vi "Scan action.vi"(8 "error in (no error)":errorcluster, 11 "SweepControl in":refnum<class "Sweep Control.lvclass">) -> (0 "error out":errorcluster, 1 "Stop?":bool, 3 "SweepControl out":refnum<class "Sweep Control.lvclass">)   [LabVIEW 2019, in "Sweep Control.lvclass"]
uses:
  Sweep Control.lvclass
  Sweep Control.lvclass/Sweep Control.ctl
  <userlib>/LevyLab/Transport/Transport/Transport.lvclass/Transport.ctl
  <userlib>/LevyLab/Instrument Framework/Instrument Types/Cryostat/Typedefs/Magnet Mode--Enum.ctl
  <userlib>/LevyLab/Transport/Control Experiment/Control Experiment.lvclass/Control Experiment.ctl
  <userlib>/LevyLab/Transport/Transport/Transport.lvclass
  <userlib>/LevyLab/Transport/Control Experiment/Control Experiment.lvclass
  <userlib>/LevyLab/Instrument Framework/Instrument Types/Lockin/Instrument.LockinAPI.lvclass
  <userlib>/LevyLab/Instrument Framework/Instrument Types/Cryostat/Instrument.Cryostat.lvclass
  <userlib>/LevyLab/Instrument Framework/Instrument Types/Strain/Instrument.Strain.lvclass
  <userlib>/LevyLab/Instrument Framework/Instrument Types/Delay Line/Instrument.DelayLine.lvclass
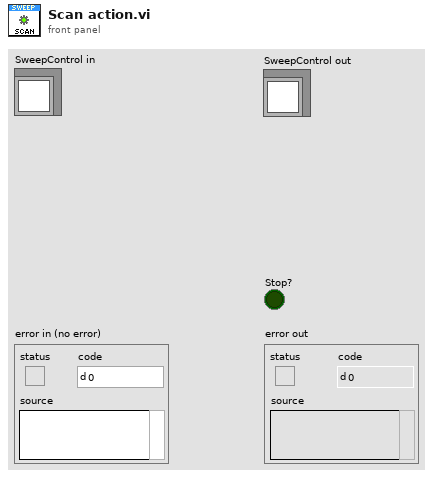
[diagram p1: front panel]
types:
  T1 = typedef "Sweep Control.lvclass/Cluster - Sweep Control.ctl" = cluster{"Start":dbl, "End":dbl, "Step":dbl, "Rate":dbl, "wait (ms/mK)":u32, "Address":string, "Priority":T2, "Scan name":T3, "Post Actions":T4[], "channel":i32}
  T2 = typedef "Sweep Control.lvclass/Enum - Priority.ctl" = enum16{"Priority 0", "Priority 1", "Priority 2", "Priority 3", "Priority 4", "Priority 5"}
  T3 = typedef "Sweep Control.lvclass/Enum - Action.ctl" = enum16{"OFF", "time", "Lockin Amplitude", "Lockin Frequency", "Lockin Bias", "Delay", "Strain", "DAQ Bias", "Magnet Field", "Temperature", "MW f1", "MW f2", "MW Amplitude1", "MW Amplitude2"}
  T4 = typedef "Sweep Control.lvclass/Enum - PostAction.ctl" = enum16{"Do Nothing", "Wait (time)", "Wait (Temperature)", "Wait (<T ; B sweep)", "Wait (Magnet)"}
  T5 = typedef "Sweep Control.lvclass/ScanParamters.ctl" = T6[]
  T6 = typedef "Sweep Control.lvclass/Cluster - ScanParamters.ctl" = cluster{"Start":dbl, "End":dbl, "Step":dbl, "Rate":dbl, "Waveform type":enum16{"linear", "triangle", "power"}, "wait (ms or K)":dbl, "Address":string, "channel":i32}
  T7 = typedef "Sweep Control.lvclass/ScanControl.ctl" = T8[]
  T8 = typedef "Sweep Control.lvclass/Cluster - ScanControl.ctl" = cluster{"Priority":T2, "Scan name":T3}
  T9 = typedef "Control Experiment.lvclass/Instrument Classes--cluster.ctl" = cluster{"DAQ":refnum<class "Instrument.LockinAPI.lvclass">, "Amplifier":refnum<class "Instrument.Amplifier.lvclass">, "Temperature":refnum<class "Instrument.Cryostat.lvclass">, "Magnet":refnum<class "Instrument.Cryostat.lvclass">, "Rotator":refnum<class "Instrument.Cryostat.lvclass">, "Level":refnum<class "Instrument.Cryostat.lvclass">, "Capacitance":refnum<class "Instrument.CBridge.lvclass">, "Delay Line":refnum<class "Instrument.DelayLine.lvclass">, "Strain Cell":refnum<class "Instrument.Strain.lvclass">, "VNA":refnum<class "Instrument.VNA.lvclass">, "Source":refnum<class "Instrument.VSource.lvclass">}
  T10 = typedef "Instrument.Cryostat.lvclass/Magnet Mode--Enum.ctl" = enum16{"Persistent", "Driven"}
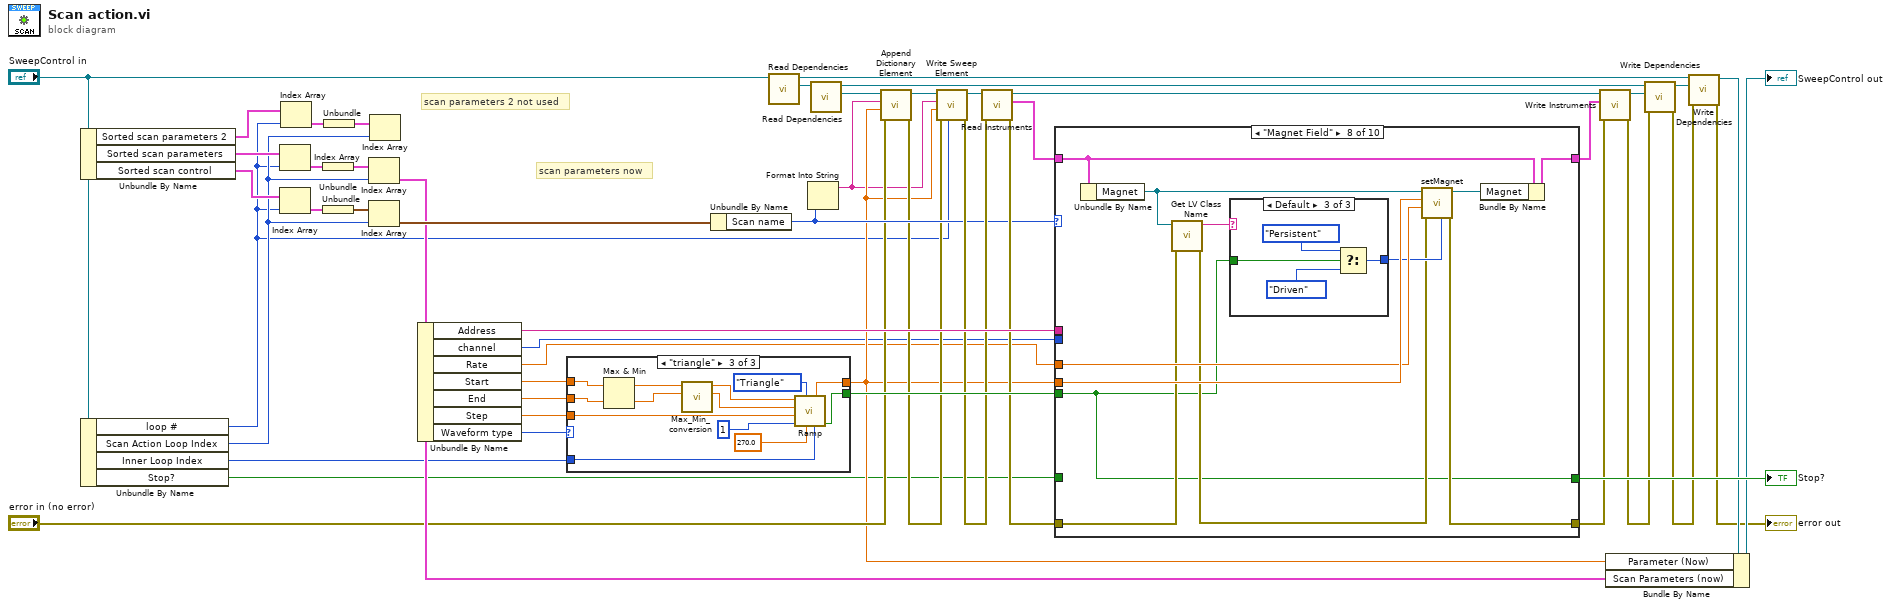
[diagram p0: block diagram]
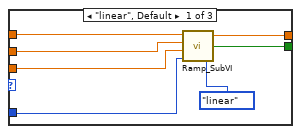
[diagram p2: hidden frame]
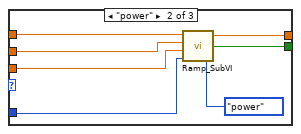
[diagram p3: hidden frame]
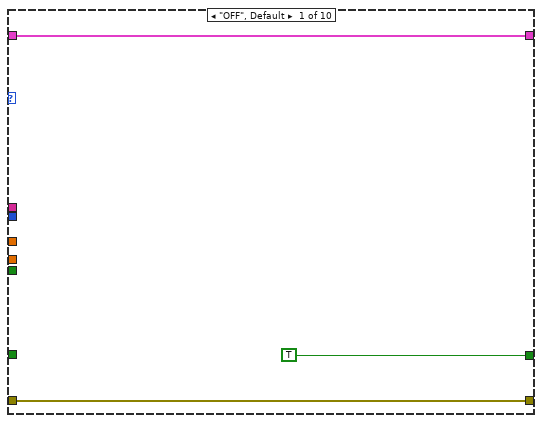
[diagram p4: hidden frame]
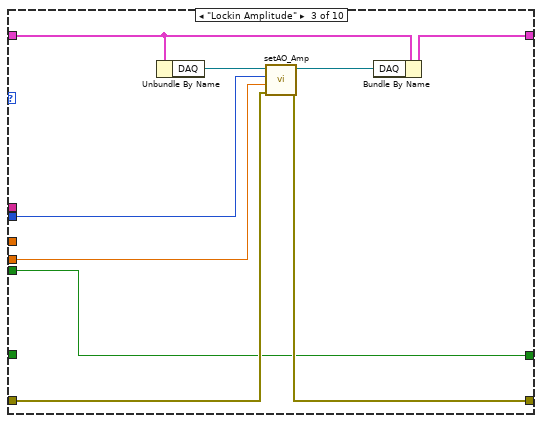
[diagram p6: hidden frame]
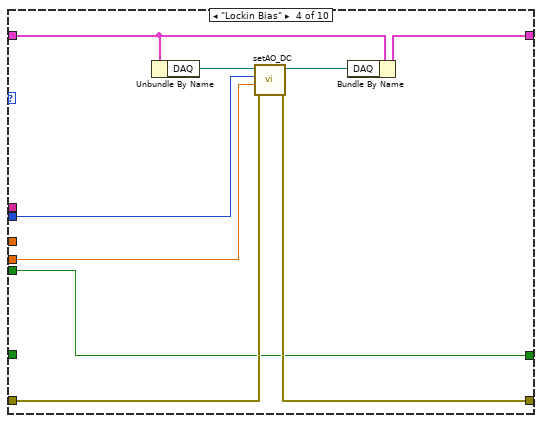
[diagram p7: hidden frame]
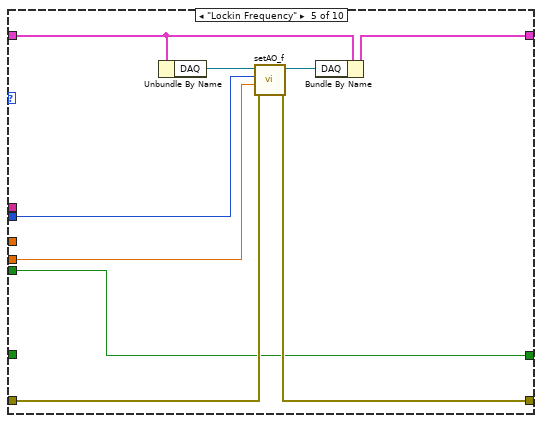
[diagram p8: hidden frame]
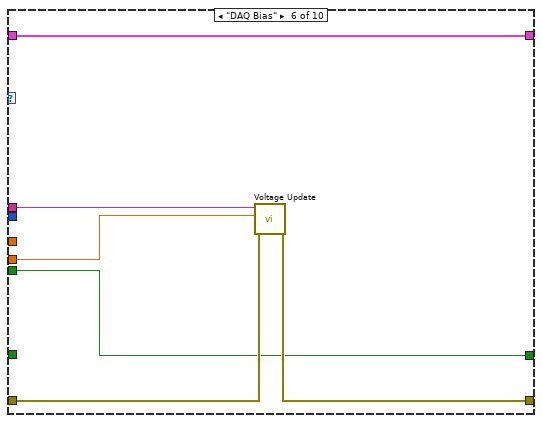
[diagram p9: hidden frame]
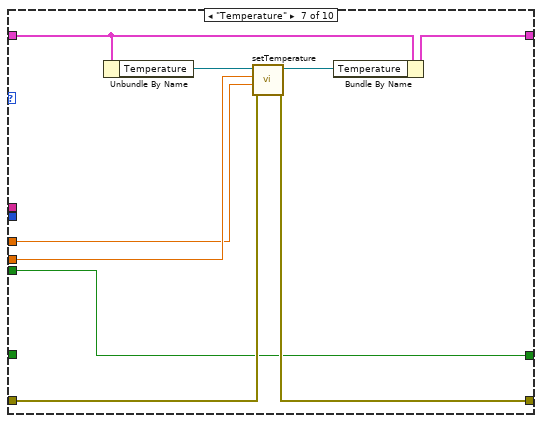
[diagram p10: hidden frame]
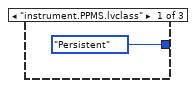
[diagram p11: hidden frame]
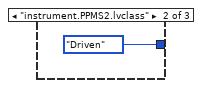
[diagram p12: hidden frame]
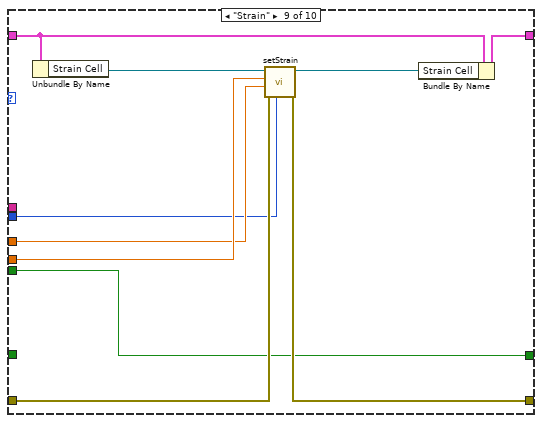
[diagram p13: hidden frame]
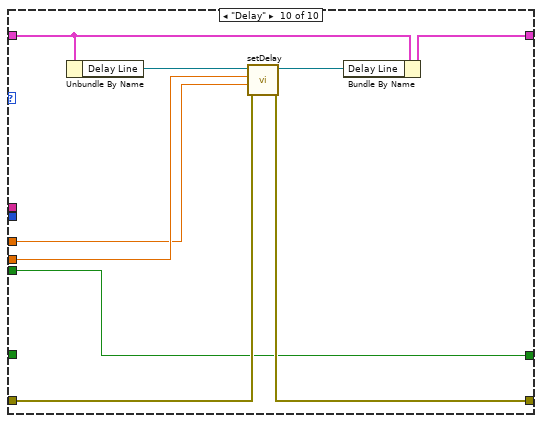
[diagram p14: hidden frame]
diagram:
  # "scan parameters 2 not used"
  # "scan parameters now"
  n1 = Unbundle By Name("SweepControl in") -> ("Sorted scan parameters 2"=w6:cluster{"Scan parameters 2":T1[]}[], "Sorted scan parameters"=w44:cluster{T5}[], "Sorted scan control"=w38:cluster{T7}[])
  n2 = Unbundle By Name("SweepControl in") -> ("loop #"=w12:i32, "Scan Action Loop Index"=w17:i32, "Inner Loop Index"=w21:i32, "Stop?"=w20:bool)
  n3 = Index Array(array=w44, index=w12) -> (element=w43:cluster{T5})
  n4 = Index Array(array=w38, index=w12) -> (element=w40:cluster{T7})
  n5 = Index Array(array=w6, index=w12) -> (element=w18:cluster{"Scan parameters 2":T1[]})
  n6 = Unbundle(w43) -> (w42:T5)
  n7 = Unbundle(w40) -> (w41:T7)
  n8 = Unbundle(w18) -> ("Scan parameters 2"=w19:T1[])
  n9 = Index Array(array=w42, index=w17) -> (element=w31:T6)
  n10 = Index Array(array=w41, index=w17) -> (element=w39:T8)
  n11 = Index Array(array=w19, index=w17) -> ()  [unwired: 1 out]
  n12 = Unbundle By Name(w31) -> ("Address"=w48:string, "channel"=w1:i32, "Rate"=w2:dbl, "Start"=w47:dbl, "End"=w37:dbl, "Step"=w36:dbl, "Waveform type"=w3:enum16{"linear", "triangle", "power"})
  n13 = case shown="\"triangle\"" w3 {
    tunnel: w47 -> [w56 w63 w67]
    tunnel: [w55 w62 w76] -> w46
    tunnel: w37 -> [w54 w61 w66]
    tunnel: w36 -> [w53 w60 w70]
    tunnel: [w52 w59 w75] -> w26
    tunnel: w21 -> [w51 w58 w71]
    frame "linear", Default {
      n14 = call <userlib>:"Ramp_SubVI.vi"("Enum"=enum16{"linear", "power"}."linear", "index"=w51, "step"=w53, "end"=w54, "start"=w56) -> ("Stop?"=w55:bool, "Numeric"=w52:dbl)
    }
    frame "power" {
      n15 = call <userlib>:"Ramp_SubVI.vi"("Enum"=enum16{"linear", "power"}."power", "index"=w58, "step"=w60, "end"=w61, "start"=w63) -> ("Stop?"=w62:bool, "Numeric"=w59:dbl)
    }
    frame "triangle" {
      n16 = Max & Min(x=w67, y=w66) -> (max(x,y)=w65:dbl, min(x,y)=w64:dbl)
      n17 = call <userlib>:"Max_Min_conversion.vi"("Min"=w64, "Max"=w65) -> ("offset"=w68:dbl, "Amplitude"=w69:dbl)  [unwired: 8 in]
      n18 = call <userlib>:"Ramp.vi"("i"=w71, "phase"=270.0, "function (ramp)"=enum16{"Ramp", "Triangle", "Sine"}."Triangle", "cycles (1,2,...)"=1, "step size"=w70, "offset"=w68, "amplitude"=w69) -> ("stop?"=w76:bool, "element"=w75:dbl)  [unwired: 2 in, 1 out]
    }
  }
  n19 = Unbundle By Name(w39) -> ("Scan name"=w30:T3)
  n20 = call <userlib>:"Read Dependencies.vi"("SweepControl in"="SweepControl in") -> ("Transport"=w8:refnum<class "Transport.lvclass">, "SweepControl out"=w7:refnum<class "Sweep Control.lvclass">)  [unwired: 8 in, 1 out]
  n21 = Format Into String(w30) -> (resulting string=w25:string)  [unwired: 3 in, 1 out]
  n22 = call <userlib>:"Read Dependencies.vi"("Transport"=w8) -> ("C.E."=w16:refnum<class "Control Experiment.lvclass">, "Transport"=w14:refnum<class "Transport.lvclass">)  [unwired: 8 in, 1 out]
  n23 = call <userlib>:"Append Dictionary Element.vi"("error in (no error)"="error in (no error)", "value"=w26, "key"=w25, "Control Experiment in"=w16) -> ("error out"=w28:errorcluster, "Control Experiment out"=w27:refnum<class "Control Experiment.lvclass">)  [unwired: 6 in]
  n24 = call <userlib>:"Write Sweep Element.vi"("loop index"=w12, "error in (no error)"=w28, "value"=w26, "key"=w25, "Control Experiment in"=w27) -> ("error out"=w34:errorcluster, "Control Experiment out"=w35:refnum<class "Control Experiment.lvclass">)  [unwired: 5 in]
  n25 = call <userlib>:"Read Instruments.vi"("error in (no error)"=w34, "Control Experiment in"=w35) -> ("error out"=w33:errorcluster, "Instruments"=w32:T9, "Control Experiment out"=w24:refnum<class "Control Experiment.lvclass">)  [unwired: 7 in]
  n26 = case shown="\"Magnet Field\"" w30 {
    tunnel: w1 -> [_ _ w89 w100 w109 _ _ _ w148 _]
    tunnel: [TRUE ("Stop?") w82 w83 w92 w101 w111 w116 w125 w144 w153] -> w49
    tunnel: w48 -> [_ _ _ _ _ w113 _ _ _ _]
    tunnel: w26 -> [_ _ w88 w99 w108 w110 w124 w135 w152 w158]
    tunnel: w46 -> [_ _ w83 w92 w101 w111 w116 w125 w144 w153]
    tunnel: w2 -> [_ _ _ _ _ _ w120 w134 w151 w157]
    tunnel: [w78 w81 w87 w98 w107 w115 w123 w136 w149 w159] -> w23
    tunnel: w32 -> [w77 w80 w85 w95 w102 w112 w118 w128 w146 w155]
    tunnel: w33 -> [w78 w81 w91 w96 w105 w114 w121 w130 w150 w160]
    tunnel: w20 -> [_ w82 _ _ _ _ _ _ _ _]
    tunnel: [w77 w80 w84 w93 w103 w112 w117 w126 w145 w154] -> w22
    frame "OFF", Default {
    }
    frame "time" {
    }
    frame "Lockin Amplitude" {
      n27 = Unbundle By Name(w85) -> ("DAQ"=w90:refnum<class "Instrument.LockinAPI.lvclass">)
      n28 = call-dynamic "setAO_Amp.vi"("error in (no error)"=w91, "Amplitude (V)"=w88, "AO Channel"=w89, "Instrument.LockinAPI in"=w90) -> ("error out"=w87:errorcluster, "Instrument.LockinAPI out"=w86:refnum<class "Instrument.LockinAPI.lvclass">)  [unwired: 6 in]
      n29 = Bundle By Name(cluster=w85, "DAQ"=w86) -> (w84:T9)
    }
    frame "Lockin Bias" {
      n30 = Unbundle By Name(w95) -> ("DAQ"=w97:refnum<class "Instrument.LockinAPI.lvclass">)
      n31 = call-dynamic "setAO_DC.vi"("error in (no error)"=w96, "DC (V)"=w99, "AO Channel"=w100, "Instrument.LockinAPI in"=w97) -> ("error out"=w98:errorcluster, "Instrument.LockinAPI out"=w94:refnum<class "Instrument.LockinAPI.lvclass">)  [unwired: 6 in]
      n32 = Bundle By Name(cluster=w95, "DAQ"=w94) -> (w93:T9)
    }
    frame "Lockin Frequency" {
      n33 = Unbundle By Name(w102) -> ("DAQ"=w106:refnum<class "Instrument.LockinAPI.lvclass">)
      n34 = call-dynamic "setAO_f.vi"("error in (no error)"=w105, "Frequency (Hz)"=w108, "AO Channel"=w109, "Instrument.LockinAPI in"=w106) -> ("error out"=w107:errorcluster, "Instrument.LockinAPI out"=w104:refnum<class "Instrument.LockinAPI.lvclass">)  [unwired: 6 in]
      n35 = Bundle By Name(cluster=w102, "DAQ"=w104) -> (w103:T9)
    }
    frame "DAQ Bias" {
      n36 = call <userlib>:"Voltage Update.vi"("error in (no error)"=w114, "Voltage Output"=w110, "Physical Channel"=w113) -> ("error out"=w115:errorcluster)  [unwired: 6 in, 2 out]
    }
    frame "Temperature" {
      n37 = Unbundle By Name(w118) -> ("Temperature"=w122:refnum<class "Instrument.Cryostat.lvclass">)
      n38 = call-dynamic "setTemperature.vi"("error in (no error)"=w121, "Rate (K/min)"=w120, "Temperature (K)"=w124, "Instrument.Cryostat in"=w122) -> ("error out"=w123:errorcluster, "Instrument.Cryostat out"=w119:refnum<class "Instrument.Cryostat.lvclass">)  [unwired: 6 in]
      n39 = Bundle By Name(cluster=w118, "Temperature"=w119) -> (w117:T9)
    }
    frame "Magnet Field" {
      n40 = Unbundle By Name(w128) -> ("Magnet"=w132:refnum<class "Instrument.Cryostat.lvclass">)
      n41 = call <vilib>:"Get LV Class Name.vi"("error in (no error)"=w130, "object"=w132) -> ("error out"=w129:errorcluster, "class name"=w131:string)  [unwired: 8 in]
      n42 = case shown="Default" w131 {
        tunnel: w125 -> [_ _ w139]
        tunnel: [Magnet_Mode--Enum."Persistent" ("Mode") Magnet_Mode--Enum."Driven" ("Mode") w142] -> w133
        frame "instrument.PPMS.lvclass" {
        }
        frame "instrument.PPMS2.lvclass" {
        }
        frame Default {
          n43 = Select(t=Magnet_Mode--Enum."Persistent" ("Mode"), s=w139, f=Magnet_Mode--Enum."Driven" ("Mode")) -> (s? t:f=w142:T10)
        }
      }
      n44 = call-dynamic "setMagnet.vi"("Mode"=w133, "error in (no error)"=w129, "Target Rate (T/min)"=w134, "Target Field (T)"=w135, "Instrument.Cryostat in"=w132) -> ("error out"=w136:errorcluster, "Instrument.Cryostat out"=w127:refnum<class "Instrument.Cryostat.lvclass">)  [unwired: 5 in]
      n45 = Bundle By Name(cluster=w128, "Magnet"=w127) -> (w126:T9)
    }
    frame "Strain" {
      n46 = Unbundle By Name(w146) -> ("Strain Cell"=w143:refnum<class "Instrument.Strain.lvclass">)
      n47 = call-dynamic "setStrain.vi"("Channel"=w148, "error in (no error)"=w150, "Slew (V/s)"=w151, "Strain (V)"=w152, "Instrument.Strain in"=w143) -> ("error out"=w149:errorcluster, "Instrument.Strain out"=w147:refnum<class "Instrument.Strain.lvclass">)  [unwired: 5 in]
      n48 = Bundle By Name(cluster=w146, "Strain Cell"=w147) -> (w145:T9)
    }
    frame "Delay" {
      n49 = Unbundle By Name(w155) -> ("Delay Line"=w161:refnum<class "Instrument.DelayLine.lvclass">)
      n50 = call-dynamic "setDelay.vi"("error in (no error)"=w160, "Rate (ps/s)"=w157, "Delay (ps)"=w158, "Instrument.Delay in"=w161) -> ("error out"=w159:errorcluster, "Instrument.Delay out"=w156:refnum<class "Instrument.DelayLine.lvclass">)  [unwired: 6 in]
      n51 = Bundle By Name(cluster=w155, "Delay Line"=w156) -> (w154:T9)
    }
  }
  "Stop?" <- w49
  n52 = call <userlib>:"Write Instruments.vi"("error in (no error)"=w23, "Instruments"=w22, "Control Experiment in"=w24) -> ("error out"=w13:errorcluster, "Control Experiment out"=w15:refnum<class "Control Experiment.lvclass">)  [unwired: 7 in]
  n53 = call <userlib>:"Write Dependencies.vi"("error in (no error)"=w13, "Control Experiment"=w15, "Transport in"=w14) -> ("error out"=w5:errorcluster, "Transport out"=w11:refnum<class "Transport.lvclass">)  [unwired: 7 in]
  n54 = call <userlib>:"Write Dependencies.vi"("error in (no error)"=w5, "Transport"=w11, "SweepControl in"=w7) -> ("error out"=→"error out":errorcluster, "SweepControl out"=w10:refnum<class "Sweep Control.lvclass">)  [unwired: 7 in]
  n55 = Bundle By Name(cluster=w10, "Parameter (Now)"=w26, "Scan Parameters (now)"=w31) -> (→"SweepControl out":refnum<class "Sweep Control.lvclass">)
